vi "PartitionBlock.vi"(8 "In_PartitionList":T1(array[cluster]), 9 "Blocks":u32[](array[numeric]), 10 "Frames":u32[](array[numeric]), 11 "Block":u32) -> (0 "Out_PartitionList":T1(array[cluster]))   [LabVIEW 2015]
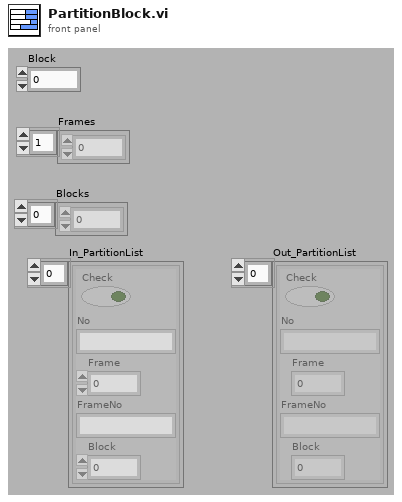
[diagram p1: front panel]
types:
  T1 = cluster{"Check":bool, "No":string, "Frame":u32, "FrameNo":string, "Block":u32}[]
  T2 = cluster{"Check":bool, "No":string, "Frame":u32, "FrameNo":string, "Block":u32}
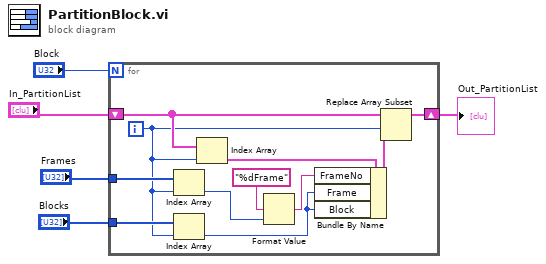
[diagram p0: block diagram]
diagram:
  n1 = for {
    N: "Block" -> [_]
    tunnel: "Blocks" -> [w11]
    shift-right: [w13] -> w3
    shift-left: "In_PartitionList" -> [w16]
    tunnel: "Frames" -> [w12]
    i -> [w7]
    n2 = Index Array(array=w12, index=w7) -> (element=w9:u32)
    n3 = Index Array(array=w11, index=w7) -> (element=w6:u32)
    n4 = Index Array(array=w16, index=w7) -> (element=w15:T2)
    n5 = Format Value(format string="%dFrame" ("形式文字列"), value (0)=w9) -> (output string=w8:string)  [unwired: 1 out]
    n6 = Bundle By Name(cluster=w15, "FrameNo"=w8, "Frame"=w6, "Block"=w6) -> (w14:T2)
    n7 = Replace Array Subset(array=w16, new element=w14, index=w7) -> (w13:T1)
  }
  "Out_PartitionList" <- w3
